vi "myRIO_BRig_RT_dataTrial_Cue2_time.vi"() -> (2 "output_Cue2_time":i32)   [LabVIEW 2014]
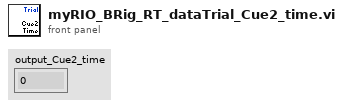
[diagram p1: front panel]
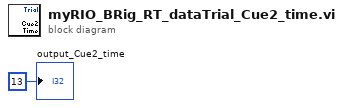
[diagram p0: block diagram]
diagram:
  "output_Cue2_time" <- 13 ("output_iBlock")
